vi "Shooter Teleop.vi"(5 "POVs":i16[](array[numeric]), 6 "Buttons":bool[](array[boolean]), 7 "Axes":dbl[](array[numeric])) -> ()   [LabVIEW 2019]
uses:
  Implementation/Shooter Operations.ctl
panel:
  in  "RPM":dbl
  in  "AL Hood":dbl
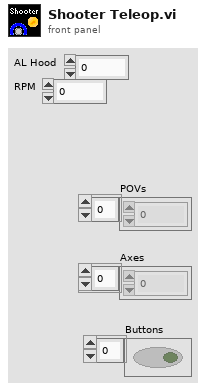
[diagram p1: front panel]
types:
  T1 = cluster{"Shooter Reset":bool, "Turret Reset":bool, "Hood Reset":bool}
  T2 = typedef "Shooter Operations.ctl" = enum16{"Reserve", "Read Current", "Immediate"}
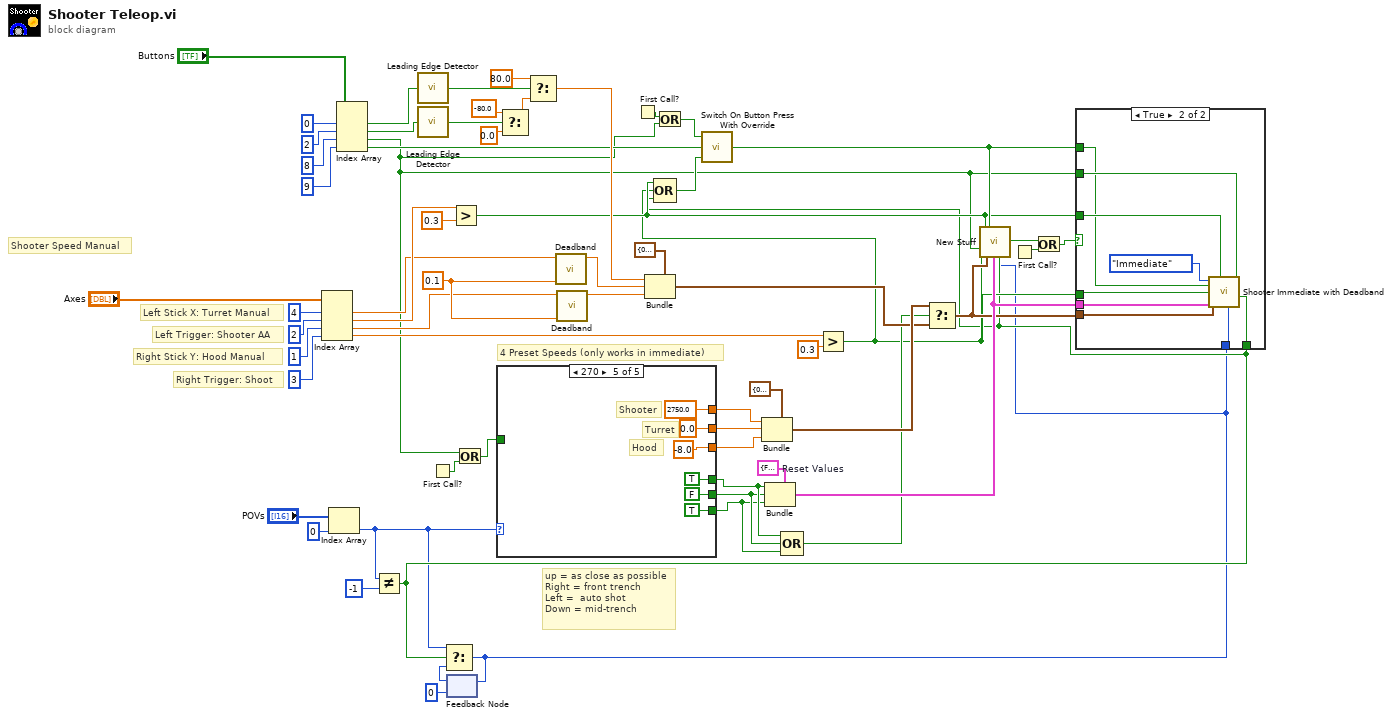
[diagram p0: block diagram]
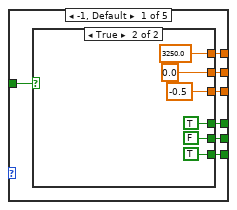
[diagram p2: hidden frame]
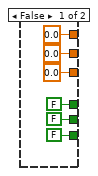
[diagram p3: hidden frame]
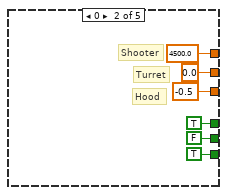
[diagram p4: hidden frame]
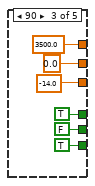
[diagram p5: hidden frame]
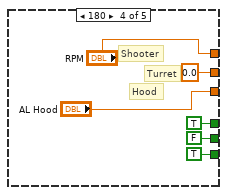
[diagram p6: hidden frame]
diagram:
  w36 = T1 {"Shooter Reset"=FALSE, "Turret Reset"=FALSE, "Hood Reset"=FALSE}  # Reset Values
  w52 = 0.1 ("Deadband")
  # "up = as close as possible\nRight = front trench\nLeft =  auto shot\nDown = mid-trench"
  # "Shooter Speed Manual"
  # "Right Stick Y: Hood Manual"
  # "Right Trigger: Shoot"
  # "Left Trigger: Shooter AA"
  # "Left Stick X: Turret Manual"
  # "4 Preset Speeds (only works in immediate)"
  n1 = Index Array(array="Axes", index #1=4 ("index"), index #2=2 ("index"), index #3=1 ("index"), index #4=3 ("index")) -> (element #1=w45:dbl, element #2=w57:dbl, element #3=w46:dbl, element #4=w53:dbl)
  n2 = Index Array(array="POVs", index=0) -> (element=w4:i16)
  n3 = Index Array(array="Buttons", index #1=0 ("index"), index #2=2 ("index"), index #3=8 ("index"), index #4=9 ("index")) -> (element #1=w48:bool, element #2=w47:bool, element #3=w7:bool, element #4=w13:bool)
  n4 = Not Equal?(x=w4, y=i16 -1) -> (x != y?=w5:bool)
  n5 = call "Leading Edge Detector.vi"("Boolean"=w48) -> ("Out"=w15:bool)
  n6 = call "Leading Edge Detector.vi"("Boolean"=w47) -> ("Out"=w20:bool)
  n7 = First Call?() -> (First Call?: T/F=w26:bool)
  n8 = feedback #1(i16 0) -> (w3:i16)
  n9 = Select(t=w4, s=w5, f=w3) -> (s? t:f=w1:i16)
  n10 = feedback-in #1(w1) -> ()
  n11 = Greater?(x=w57, y=0.3) -> (0:w10:bool)
  n12 = Or(x=w7, y=w26) -> (x .or. y?=w27:bool)
  n13 = case shown="270" w4 {
    tunnel: [w69 4500.0 3500.0 ("RPM") "RPM" 2750.0] -> w40
    tunnel: [w68 0.0 0.0 ("Turret") 0.0 0.0] -> w39
    tunnel: [w67 -0.5 -14.0 ("AL Hood") "AL Hood" -8.0 ("AL Hood")] -> w38
    tunnel: w27 -> [w70 _ _ _ _]
    tunnel: [w66 TRUE TRUE TRUE TRUE] -> w31
    tunnel: [w65 FALSE FALSE FALSE FALSE] -> w30
    tunnel: [w64 TRUE TRUE TRUE TRUE] -> w29
    frame -1, Default {
      n14 = case shown="True" w70 {
        tunnel: [0.0 3250.0] -> w69
        tunnel: [0.0 0.0] -> w68
        tunnel: [0.0 -0.5] -> w67
        tunnel: [FALSE TRUE] -> w66
        tunnel: [FALSE FALSE] -> w65
        tunnel: [FALSE TRUE] -> w64
        frame False {
        }
        frame True {
        }
      }
    }
    frame 0 {
      # "Turret"
      # "Hood"
      # "Shooter"
    }
    frame 90 {
    }
    frame 180 {
      # "Turret"
      # "Hood"
      # "Shooter"
    }
    frame 270 {
      # "Turret"
      # "Hood"
      # "Shooter"
    }
  }
  n15 = Select(t=-80.0, s=w20, f=0.0) -> (s? t:f=w19:dbl)
  n16 = Select(t=80.0, s=w15, f=w19) -> (s? t:f=w43:dbl)
  n17 = call "Deadband.vi"("Deadband"=w52, "Input"=w45) -> ("f"=w42:dbl)  [unwired: 9 in]
  n18 = call "Deadband.vi"("Deadband"=w52, "Input"=w46) -> ("f"=w41:dbl)  [unwired: 9 in]
  n19 = First Call?() -> (First Call?: T/F=w8:bool)
  n20 = Bundle(cluster=cluster{"Shooter":dbl, "Turret":dbl, "Hood":dbl} {"Shooter"=0.0, "Turret"=0.0, "Hood"=0.0} ("Setpoints"), "Shooter"=w43, "Turret"=w42, "Hood"=w41) -> (w33:cluster{"Shooter":dbl, "Turret":dbl, "Hood":dbl})
  n21 = Or(x=w8, y=w7) -> (x .or. y?=w6:bool)
  n22 = Bundle(cluster=cluster{"Shooter":dbl, "Turret":dbl, "Hood":dbl} {"Shooter"=0.0, "Turret"=0.0, "Hood"=0.0} ("Setpoints"), "Shooter"=w40, "Turret"=w39, "Hood"=w38) -> (w34:cluster{"Shooter":dbl, "Turret":dbl, "Hood":dbl})
  n23 = Bundle(cluster=w36, "Shooter Reset"=w31, "Turret Reset"=w30, "Hood Reset"=w29) -> (w35:T1)
  n24 = Compound Arithmetic op=OR(w31, w30, w29) -> (w28:bool)
  n25 = Greater?(x=w53, y=0.3) -> (0:w9:bool)
  n26 = Compound Arithmetic op=OR(w10, w9, w5) -> (w11:bool)
  n27 = call "Switch On Button Press With Override.vi"("Override False"=w11, "Button"=w13, "Override True"=w6) -> ("Output"=w12:bool)
  n28 = Select(t=w34, s=w28, f=w33) -> (s? t:f=w32:cluster{"Shooter":dbl, "Turret":dbl, "Hood":dbl})
  n29 = call "New Stuff.vi"("Variant 15"=w7, "Variant 7"=w9, "Variant 5"=w10, "Variant 14"=w32, "Variant 12"=w12, "Variant 11"=w5, "Variant 6"=w35, "Variant 9"=w1) -> ("x != y?"=w23:bool)  [unwired: 19 in]
  n30 = First Call?() -> (First Call?: T/F=w21:bool)
  n31 = Or(x=w23, y=w21) -> (x .or. y?=w22:bool)
  n32 = case shown="True" w22 {
    tunnel: w35 -> [_ w115]
    tunnel: w10 -> [_ w114]
    tunnel: w32 -> [_ w112]
    tunnel: w9 -> [_ w111]
    tunnel: w7 -> [_ w110]
    tunnel: w5 -> [_ w109]
    tunnel: w12 -> [_ w108]
    tunnel: w1 -> [_ w107]
    frame False {
    }
    frame True {
      n33 = call "Shooter Immediate with Deadband.vi"("POVs"=w109, "Shoot"=w111, "Reset"=w110, "Shot Position"=w107, "Auto-Shot"=w114, "Reset Values"=w115, "Setpoints"=w112, "Homing?"=w108, "Operation"=Shooter_Operations."Immediate") -> ()  [unwired: 1 in, 1 out]
    }
  }
